vi "save_config_svi.vi"(0 "Refnum VISA en entrée":refnum<visa-resource-name>, 1 "EXPT":dbl, 2 "Nstart":u32, 3 "config Name":string, 4 "BETWEEN_PAT":u32, 5 "BIN":u16, 6 "NPAT":u32, 8 "Non":u32, 9 "ROMODE":u32, 10 "SOFT_VERSION":string, 11 "Camera Model":string, 12 "Noff":u32, 13 "Camera Serial":string, 14 "Config Directory":path, 15 "Version":string, 16 "USED_FILTERS":u8[](array[numeric]), 17 "STAGE_SPEED":dbl, 18 "USED_LEDS":bool[][](array[boolean]), 19 "XYPOS":T1, 26 "BETWEEN_SCAN":u32, 27 "NSCAN":u32) -> ()   [LabVIEW 2013]
uses:
  <vilib>/Analysis/Matrix/Datatypes/RealMatrix.ctl
  <vilib>/Analysis/Matrix/NI_Matrix.lvlib
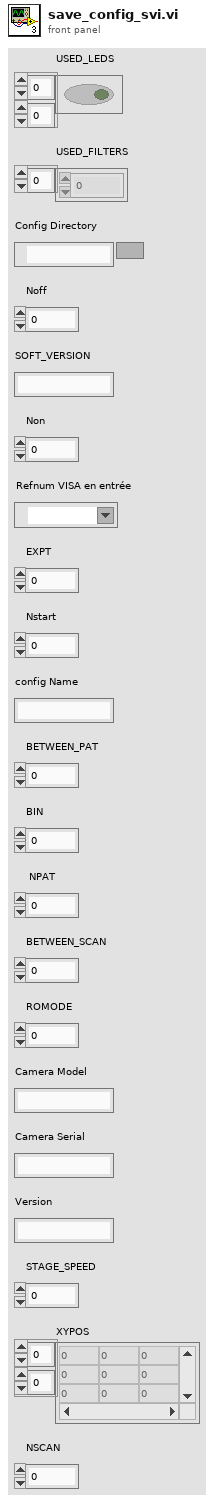
[diagram p1: front panel]
types:
  T1 = typedef "NI_Matrix.lvlib/RealMatrix.ctl" = dbl[][]
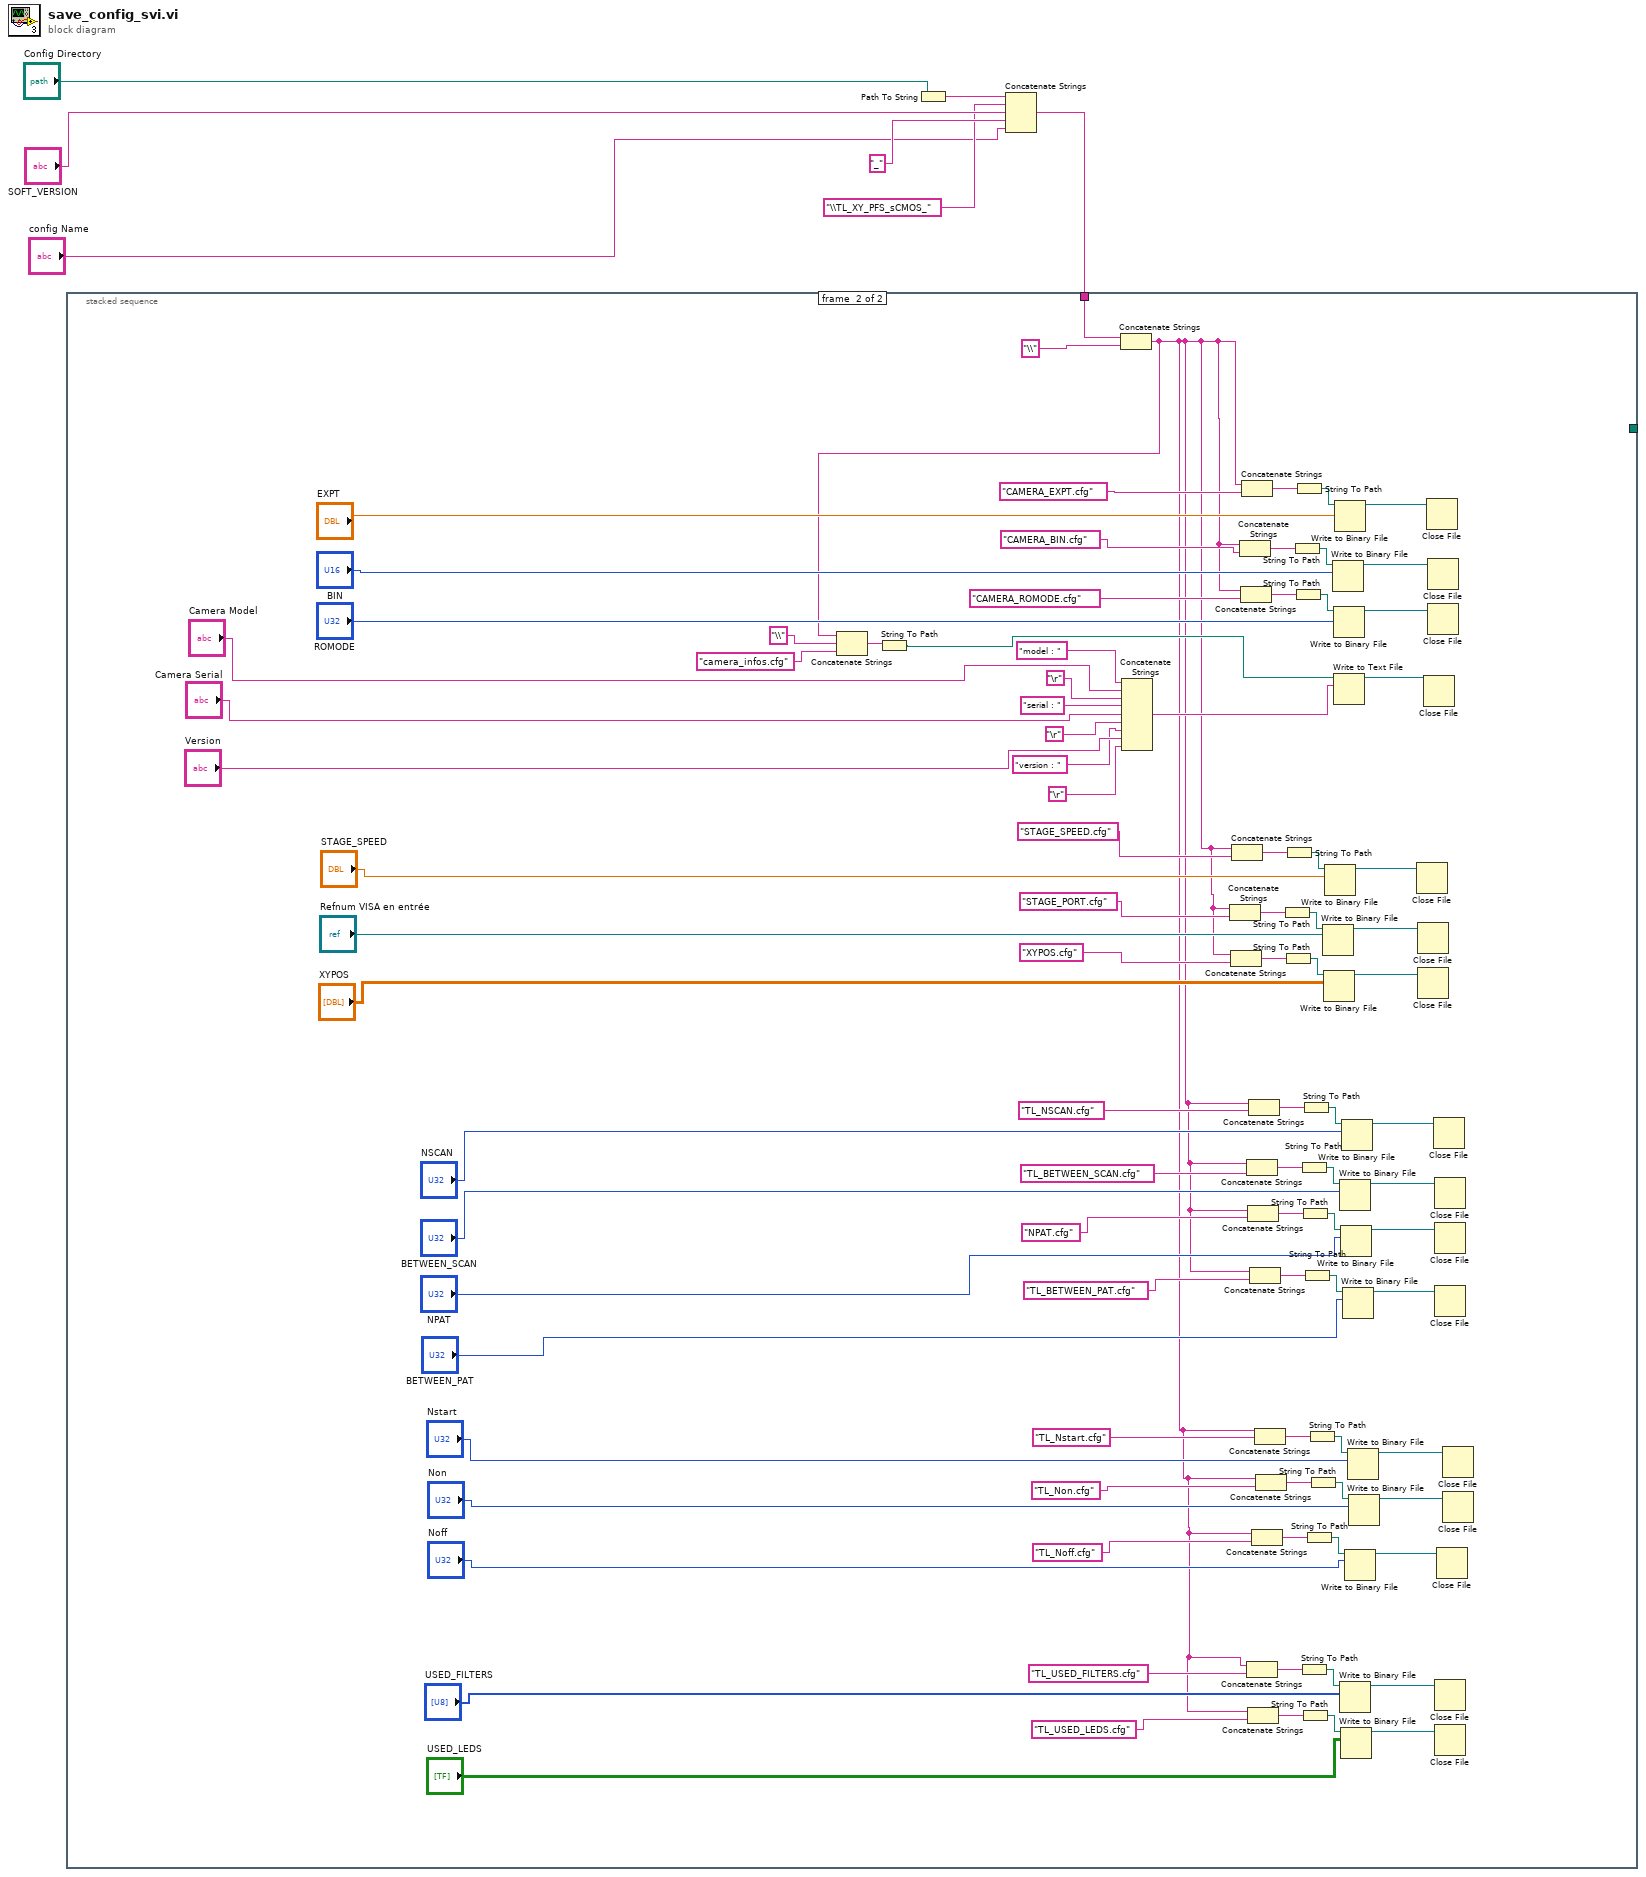
[diagram p0: block diagram]
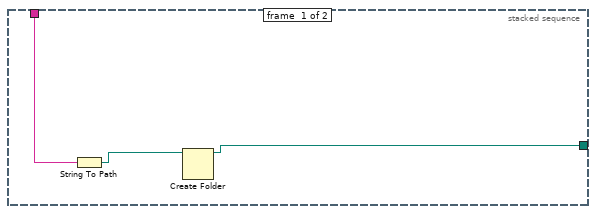
[diagram p2: hidden frame]
diagram:
  n1 = Path To String(path="Config Directory") -> (string=w2:string)
  n2 = Concatenate Strings(w2, "\\TL_XY_PFS_sCMOS_", "SOFT_VERSION", "_", "config Name") -> (w7:string)
  n3 = stacked-sequence {
    tunnel: w7 -> [w9 w13]
    tunnel: [w8 _] -> _
    frame #0 {
      n4 = String To Path(string=w9) -> (path=w10:path)
      n5 = Create Folder(path (use dialog)=w10) -> (created path=w8:path)  [unwired: 2 in, 2 out]
    }
    frame #1 {
      n6 = Concatenate Strings(w13, "\\") -> (w11:string)
      n7 = Concatenate Strings(w11, "\\", "camera_infos.cfg") -> (w100:string)
      n8 = String To Path(string=w100) -> (path=w103:path)
      n9 = Concatenate Strings("model : ", "Camera Model", "\r", "serial : ", "Camera Serial", "\r", "version : ", "Version", "\r") -> (w35:string)
      n10 = Concatenate Strings(w11, "STAGE_PORT.cfg") -> (w41:string)
      n11 = Concatenate Strings(w11, "XYPOS.cfg") -> (w42:string)
      n12 = Concatenate Strings(w11, "STAGE_SPEED.cfg") -> (w40:string)
      n13 = Concatenate Strings(w11, "CAMERA_BIN.cfg") -> (w18:string)
      n14 = Concatenate Strings(w11, "CAMERA_ROMODE.cfg") -> (w23:string)
      n15 = Concatenate Strings(w11, "CAMERA_EXPT.cfg") -> (w17:string)
      n16 = Concatenate Strings(w11, "TL_BETWEEN_SCAN.cfg") -> (w56:string)
      n17 = Concatenate Strings(w11, "TL_USED_FILTERS.cfg") -> (w74:string)
      n18 = Concatenate Strings(w11, "NPAT.cfg") -> (w57:string)
      n19 = Concatenate Strings(w11, "TL_USED_LEDS.cfg") -> (w75:string)
      n20 = Concatenate Strings(w11, "TL_NSCAN.cfg") -> (w55:string)
      n21 = Concatenate Strings(w11, "TL_BETWEEN_PAT.cfg") -> (w64:string)
      n22 = Concatenate Strings(w11, "TL_Noff.cfg") -> (w73:string)
      n23 = Concatenate Strings(w11, "TL_Nstart.cfg") -> (w65:string)
      n24 = Concatenate Strings(w11, "TL_Non.cfg") -> (w66:string)
      n25 = String To Path(string=w41) -> (path=w44:path)
      n26 = String To Path(string=w42) -> (path=w45:path)
      n27 = String To Path(string=w40) -> (path=w43:path)
      n28 = String To Path(string=w18) -> (path=w19:path)
      n29 = String To Path(string=w23) -> (path=w24:path)
      n30 = String To Path(string=w17) -> (path=w15:path)
      n31 = String To Path(string=w56) -> (path=w59:path)
      n32 = String To Path(string=w74) -> (path=w77:path)
      n33 = String To Path(string=w57) -> (path=w60:path)
      n34 = String To Path(string=w75) -> (path=w78:path)
      n35 = String To Path(string=w55) -> (path=w58:path)
      n36 = String To Path(string=w64) -> (path=w67:path)
      n37 = String To Path(string=w73) -> (path=w76:path)
      n38 = String To Path(string=w65) -> (path=w68:path)
      n39 = String To Path(string=w66) -> (path=w69:path)
      n40 = Write to Binary File(file (use dialog)=w44, data="Refnum VISA en entrée") -> (refnum out=w47:refnum<file>)  [unwired: 4 in, 2 out]
      n41 = Write to Binary File(file (use dialog)=w45, data="XYPOS") -> (refnum out=w48:refnum<file>)  [unwired: 4 in, 2 out]
      n42 = Write to Binary File(file (use dialog)=w43, data="STAGE_SPEED") -> (refnum out=w46:refnum<file>)  [unwired: 4 in, 2 out]
      n43 = Write to Binary File(file (use dialog)=w19, data="BIN") -> (refnum out=w37:refnum<file>)  [unwired: 4 in, 2 out]
      n44 = Write to Binary File(file (use dialog)=w24, data="ROMODE") -> (refnum out=w38:refnum<file>)  [unwired: 4 in, 2 out]
      n45 = Write to Text File(file (use dialog)=w103, text=w35) -> (refnum out=w39:refnum<file>)  [unwired: 2 in, 2 out]
      n46 = Write to Binary File(file (use dialog)=w15, data="EXPT") -> (refnum out=w36:refnum<file>)  [unwired: 4 in, 2 out]
      n47 = Write to Binary File(file (use dialog)=w59, data="BETWEEN_SCAN") -> (refnum out=w62:refnum<file>)  [unwired: 4 in, 2 out]
      n48 = Write to Binary File(file (use dialog)=w77, data="USED_FILTERS") -> (refnum out=w80:refnum<file>)  [unwired: 4 in, 2 out]
      n49 = Write to Binary File(file (use dialog)=w60, data="NPAT") -> (refnum out=w63:refnum<file>)  [unwired: 4 in, 2 out]
      n50 = Write to Binary File(file (use dialog)=w78, data="USED_LEDS") -> (refnum out=w81:refnum<file>)  [unwired: 4 in, 2 out]
      n51 = Write to Binary File(file (use dialog)=w58, data="NSCAN") -> (refnum out=w61:refnum<file>)  [unwired: 4 in, 2 out]
      n52 = Write to Binary File(file (use dialog)=w67, data="BETWEEN_PAT") -> (refnum out=w70:refnum<file>)  [unwired: 4 in, 2 out]
      n53 = Write to Binary File(file (use dialog)=w76, data="Noff") -> (refnum out=w79:refnum<file>)  [unwired: 4 in, 2 out]
      n54 = Write to Binary File(file (use dialog)=w68, data="Nstart") -> (refnum out=w71:refnum<file>)  [unwired: 4 in, 2 out]
      n55 = Write to Binary File(file (use dialog)=w69, data="Non") -> (refnum out=w72:refnum<file>)  [unwired: 4 in, 2 out]
      n56 = Close File(refnum=w46) -> ()  [unwired: 1 in, 2 out]
      n57 = Close File(refnum=w47) -> ()  [unwired: 1 in, 2 out]
      n58 = Close File(refnum=w48) -> ()  [unwired: 1 in, 2 out]
      n59 = Close File(refnum=w39) -> ()  [unwired: 1 in, 2 out]
      n60 = Close File(refnum=w36) -> ()  [unwired: 1 in, 2 out]
      n61 = Close File(refnum=w37) -> ()  [unwired: 1 in, 2 out]
      n62 = Close File(refnum=w38) -> ()  [unwired: 1 in, 2 out]
      n63 = Close File(refnum=w61) -> ()  [unwired: 1 in, 2 out]
      n64 = Close File(refnum=w62) -> ()  [unwired: 1 in, 2 out]
      n65 = Close File(refnum=w63) -> ()  [unwired: 1 in, 2 out]
      n66 = Close File(refnum=w70) -> ()  [unwired: 1 in, 2 out]
      n67 = Close File(refnum=w80) -> ()  [unwired: 1 in, 2 out]
      n68 = Close File(refnum=w81) -> ()  [unwired: 1 in, 2 out]
      n69 = Close File(refnum=w79) -> ()  [unwired: 1 in, 2 out]
      n70 = Close File(refnum=w71) -> ()  [unwired: 1 in, 2 out]
      n71 = Close File(refnum=w72) -> ()  [unwired: 1 in, 2 out]
    }
  }
